vi "setUp.vi"(8 "error in (no error)":errorcluster, 11 "reference in":refnum<class "Test Network Stream Transmission.lvclass">) -> (0 "error out":errorcluster, 3 "reference out":refnum<class "Test Network Stream Transmission.lvclass">)   [LabVIEW 2020, in "Test Network Stream Transmission.lvclass"]
doc: "setUp runs prior to the test method during test execution. Use this method to initialize any object data required by your tests."
uses:
  Test Network Stream Transmission.lvclass
  <vilib>/addons/_JKI Toolkits/VI Tester/TestCase.llb/TestCase.lvclass
  Source/Protocols/Network Stream Strategy/Network Stream Initiator/Network Stream Initiator.lvclass
  Source/Ciphers/AES/AES.lvclass
  Source/Ciphers/AES/Ton Plomp Encryption/AES-Modes.ctl
  Source/Ciphers/AES/Ton Plomp Encryption/Encryption.lvlib
  Source/Abstract Classes/Message Stream/Message Stream.lvclass
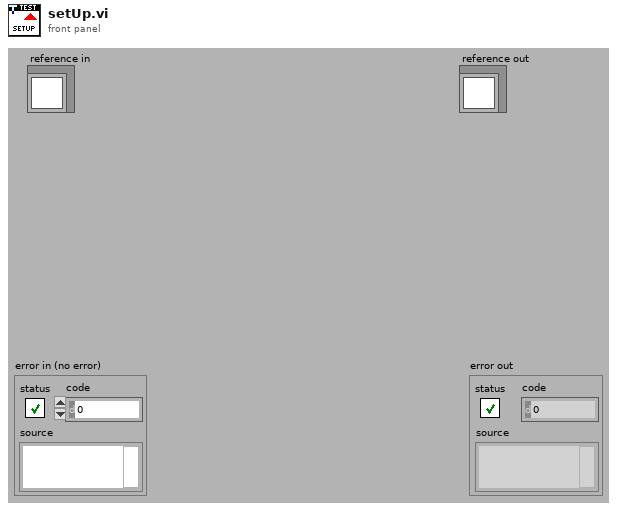
[diagram p1: front panel]
types:
  T1 = typedef "Encryption.lvlib/AES-Modes.ctl" = enum16{"ECB", "CBC", "CFB128", "OFB"}
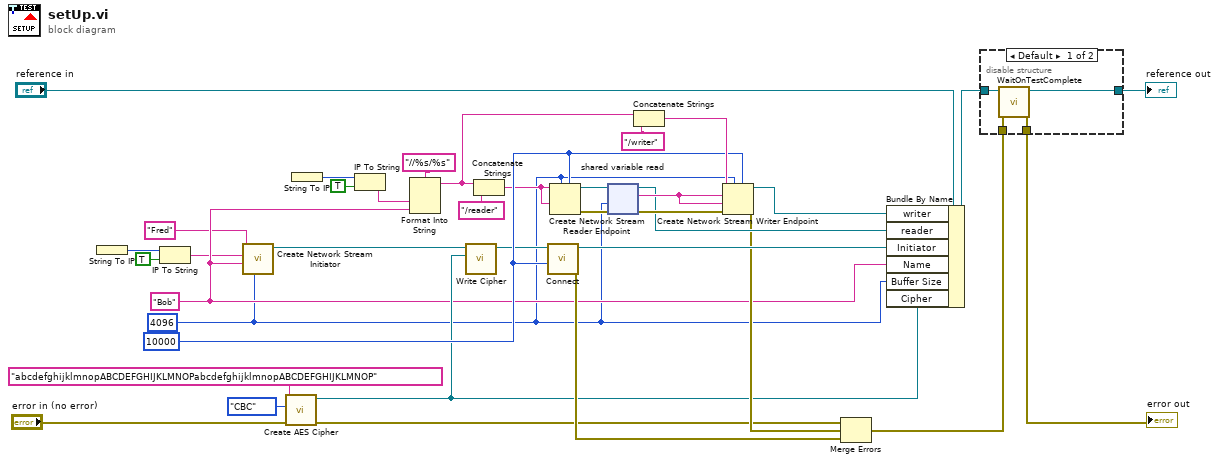
[diagram p0: block diagram]
diagram:
  w23 = 10000 ("timeout")
  w1 = 4096 ("Buffer Size")
  w4 = "Bob" ("Remote Name")
  n1 = String To IP() -> (0:w33:u32)  [unwired: 1 in]
  n2 = IP To String(1:TRUE ("dot notation? (F)"), 2:w33) -> (0:w3:string)
  n3 = call "Create Network Stream Initiator.vi"("Buffer Size"=w1, "Remote Name"=w4, "Remote Address"=w3, "Name"="Fred") -> ("Network Stream Initiator out"=w31:refnum<class "Network Stream Initiator.lvclass">)  [unwired: 7 in]
  n4 = call "Create AES Cipher.vi"("error in (no error)"="error in (no error)", "Operation Mode"=AES-Modes."CBC", "Cipher Key"="abcdefghijklmnopABCDEFGHIJKLMNOPabcdefghijklmnopABCDEFGHIJKLMNOP") -> ("error out"=w6:errorcluster, "AES out"=w5:refnum<class "AES.lvclass">)  [unwired: 7 in]
  n5 = String To IP() -> (0:w18:u32)  [unwired: 1 in]
  n6 = IP To String(1:TRUE ("dot notation? (F)"), 2:w18) -> (0:w20:string)
  n7 = Format Into String(format string="//%s/%s", w20, w4) -> (resulting string=w29:string)  [unwired: 2 in, 1 out]
  n8 = call "Write Cipher.vi"("Cipher"=w5, "Message Stream in"=w31) -> ("Message Stream out"=w10:refnum<class "Network Stream Initiator.lvclass">)  [unwired: 9 in]
  n9 = Concatenate Strings(w29, "/reader" ("format string")) -> (w21:string)
  n10 = call-dynamic "Connect.vi"("timeout"=w23, "Network Stream Initiator in"=w10) -> ("error out"=w12:errorcluster, "Network Stream Initiator out"=w16:refnum<class "Network Stream Initiator.lvclass">)  [unwired: 8 in]
  n11 = Create Network Stream Reader Endpoint(5:w23, 7:w1, 9:w21, 11:w21) -> (0:w24:errorcluster, 3:w25:refnum<k21>)  [unwired: 3 in]
  n12 = shared-variable-read(w25, w24, w1) -> (w15:refnum<k21>, w26:errorcluster, w27:string)  [unwired: 1 out]
  n13 = Concatenate Strings(w29, "/writer" ("format string")) -> (w30:string)
  n14 = Create Network Stream Writer Endpoint(5:w23, 7:w1, 8:w26, 9:w27, 10:w27, 11:w30) -> (0:w11:errorcluster, 3:w14:refnum<k21>)  [unwired: 1 in]
  n15 = Merge Errors(w6, w11, w12) -> (w13:errorcluster)
  n16 = Bundle By Name(cluster="reference in", "writer"=w14, "reader"=w15, "Initiator"=w16, "Name"=w4, "Buffer Size"=w1, "Cipher"=w5) -> (w34:refnum<class "Test Network Stream Transmission.lvclass">)
  n17 = disable-structure shown="Default" {
    disable-tunnel: w13 -> [w41 w42]
    disable-tunnel: [w40 w42] -> w37
    disable-tunnel: [w39 w43] -> w35
    disable-tunnel: w34 -> [w38 w43]
    frame condition #0 (active) {
      n18 = call <vilib>:"WaitOnTestComplete.vi"("error in (no error)"=w41, "TestCase in"=w38) -> ("error out"=w40:errorcluster, "TestCase out"=w39:refnum<class "Test Network Stream Transmission.lvclass">)  [unwired: 8 in]
    }
    frame condition #1 {
    }
  }
  "error out" <- w37
  "reference out" <- w35
